vi "IP.vi"() -> ()   [LabVIEW 2015]
panel:
  out "net address":u32
  out "name":string
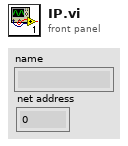
[diagram p1: front panel]
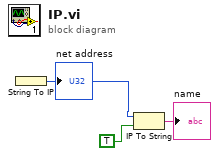
[diagram p0: block diagram]
diagram:
  n1 = String To IP() -> (0:w3:u32)  [unwired: 1 in]
  "net address" <- w3
  n2 = IP To String(1:TRUE, 2:w3) -> (0:→"name":string)
